vi "Enable Embedded Data Logger Custom Device.vi"(8 "error in":errorcluster, 11 "embedded data logger in":T1 format="%.0x") -> (0 "error out":errorcluster, 3 "embedded data logger out":T1 format="%.0x")   [LabVIEW 2027, in "Embedded Data Logger Scripting.lvlib"]
uses:
  Embedded Data Logger Scripting.lvlib
  <vilib>/NI VeriStand/Custom Device API/Custom Device API.lvlib
  Shared/Constants.vi
  Shared/Embedded Data Logger Shared.lvlib
  C:/NetCore/niveristand-embedded-data-logger-custom-device/Source/Scripting/Custom Device/Enable Embedded Data Logger Custom Device.vi/NationalInstruments.VeriStand.SystemDefinitionAPI
  NationalInstruments.VeriStand.SystemDefinitionAPI
  <vilib>/NI VeriStand/Custom Device API/Custom Device Item Ref.ctl
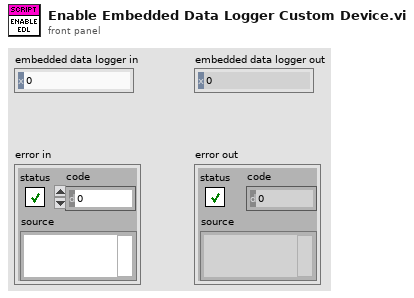
[diagram p1: front panel]
types:
  T1 = typedef "Custom Device API.lvlib/Custom Device Item Ref.ctl" = u64
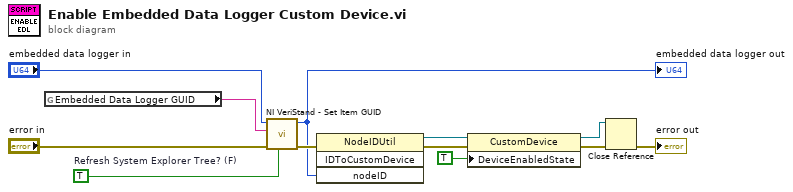
[diagram p0: block diagram]
diagram:
  w12 = TRUE  # Refresh System Explorer Tree? (F)
  n1 = global read "Constants.vi" "Embedded Data Logger GUID"() -> (w11:string)
  n2 = call <vilib>:"NI VeriStand - Set Item GUID.vi"("Refresh System Explorer Tree? (F)"=w12, "error in (no error)"="error in", "GUID"=w11, "Item Ref in"="embedded data logger in") -> ("error out"=w3:errorcluster, "Item Ref out"=w1:T1)  [unwired: 6 in]
  "embedded data logger out" <- w1
  n3 = invoke class="NodeIDUtil" method="IDToCustomDevice"(error in=w3, "nodeID"=w1) -> (error out=w6:errorcluster, "IDToCustomDevice"=w8:refnum<k39>)  [unwired: 2 in, 2 out]
  n4 = property class="CustomDevice"(reference=w8, error in=w6, "DeviceEnabledState"=TRUE) -> (reference out=w4:refnum<k39>, error out=w5:errorcluster)
  n5 = Close Reference(reference=w4, error in (no error)=w5) -> (error out=→"error out":errorcluster)
